vi "Stop Core.vi"(10 "final error code":i32, 11 "Controller in":refnum<class "Controller.lvclass">) -> (3 "Controller out":refnum<class "Controller.lvclass">)   [LabVIEW 2013, in "SET Project Editor.lvlib" / "Controller.lvclass"]
doc: "(<B>Filename</B>: Actor Framework.lvlib:Actor.lvclass:Stop Core.vi)\n\nDefines what the actor does before it stops. Use the <B>final error code</B> input to determine whether the actor shut down in response to an error.\n\nBy default, this method does nothing. A descendant class may override it to define behavior, such as shutting down any processes the actor initiated in its override of the Actor Core method."
uses:
  Controller.lvclass
  Controller.lvclass/Controller.ctl
  SET Project Data/Project Data Class/Project Data.lvclass
  <vilib>/ActorFramework/Message Enqueuer/Message Enqueuer.lvclass/Message Enqueuer.ctl
  UI Actor/UI Actor.lvclass
  <vilib>/ActorFramework/Message Enqueuer/Enqueue.vi
  <vilib>/ActorFramework/Message Priority Queue/Priority Enqueue.vi
  <vilib>/ActorFramework/Stop Msg/Stop Msg.lvclass
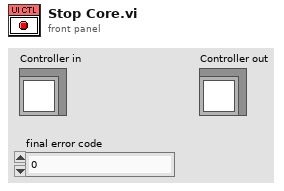
[diagram p1: front panel]
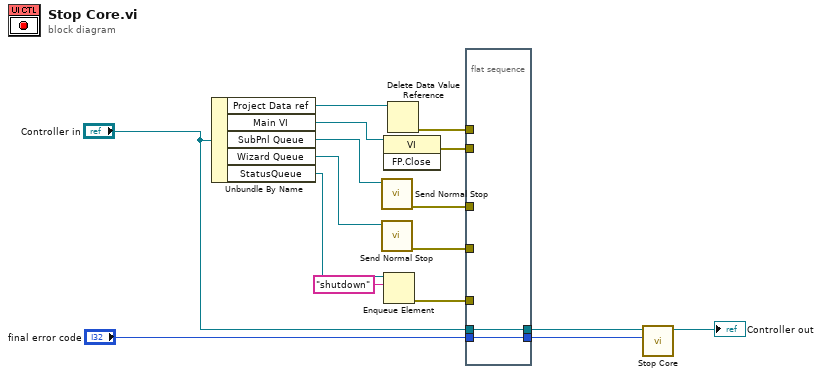
[diagram p0: block diagram]
diagram:
  n1 = Unbundle By Name("Controller in") -> ("Project Data ref"=w9:refnum<data-value>, "Main VI"=w11:refnum<vi>, "SubPnl Queue"=w7:refnum<class "Message Enqueuer.lvclass">, "Wizard Queue"=w5:refnum<class "Message Enqueuer.lvclass">, "StatusQueue"=w3:refnum<queue>)
  n2 = call <vilib>:"Send Normal Stop.vi"("Message Enqueuer"=w7) -> ("error out"=w6:errorcluster)  [unwired: 10 in]
  n3 = call <vilib>:"Send Normal Stop.vi"("Message Enqueuer"=w5) -> ("error out"=w4:errorcluster)  [unwired: 10 in]
  n4 = invoke class="VI" method="FP.Close"(reference=w11) -> (error out=w10:errorcluster)  [unwired: 2 in, 2 out]
  n5 = Enqueue Element(queue=w3, element="shutdown") -> (error out=w1:errorcluster)  [unwired: 2 in, 2 out]
  n6 = Delete Data Value Reference(data value reference=w9) -> (error out=w8:errorcluster)  [unwired: 1 in, 1 out]
  n7 = flat-sequence {
    tunnel: "final error code" -> [w18]
    tunnel: [w18] -> w14
    tunnel: [w17] -> w12
    tunnel: "Controller in" -> [w17]
    tunnel: w10 -> [_]
    tunnel: w8 -> [_]
    tunnel: w6 -> [_]
    tunnel: w4 -> [_]
    tunnel: w1 -> [_]
    frame #0 {
    }
  }
  n8 = call-parent "Stop Core.vi"("final error code"=w14, "UI Actor in"=w12) -> ("UI Actor out"=→"Controller out":refnum<class "Controller.lvclass">)  [unwired: 9 in]
